vi "4155C Sample Config SMUs FPP v2.0.vi"(2 "FPP - Probe 2":u32(ring)=3 items=["SMU1  ", "SMU2  ", "SMU3  ", "SMU4  ", "SMU5  ", "SMU6  "], 4 "FPP - Probe 1":u32(ring) items=["SMU1  ", "SMU2  ", "SMU3  ", "SMU4  ", "SMU5  ", "SMU6  "], 5 "FPP - Drain":u32(ring)=1 items=["SMU1  ", "SMU2  ", "SMU3  ", "SMU4  ", "SMU5  ", "SMU6  "], 6 "FPP - Gate":u32(ring)=2 items=["SMU1  ", "SMU2  ", "SMU3  ", "SMU4  ", "SMU5  ", "SMU6  "], 7 "FPP - Source":u32(ring) items=["VSU1  ", "VSU2  "], 8 "error in (no error)":errorcluster, 9 "Drain Standby":bool, 10 "Gate Standby":bool, 11 "VISA resource name in":refnum<visa-resource-name>) -> (0 "error out":errorcluster, 3 "VISA Resource Name out":refnum<visa-resource-name>)   [LabVIEW 2016]
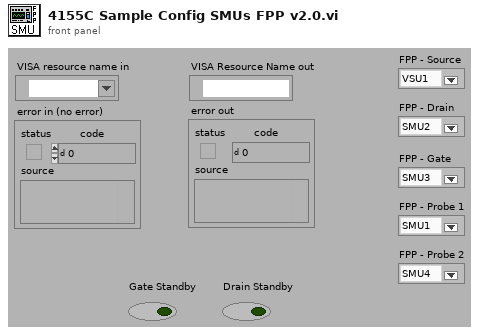
[diagram p1: front panel]
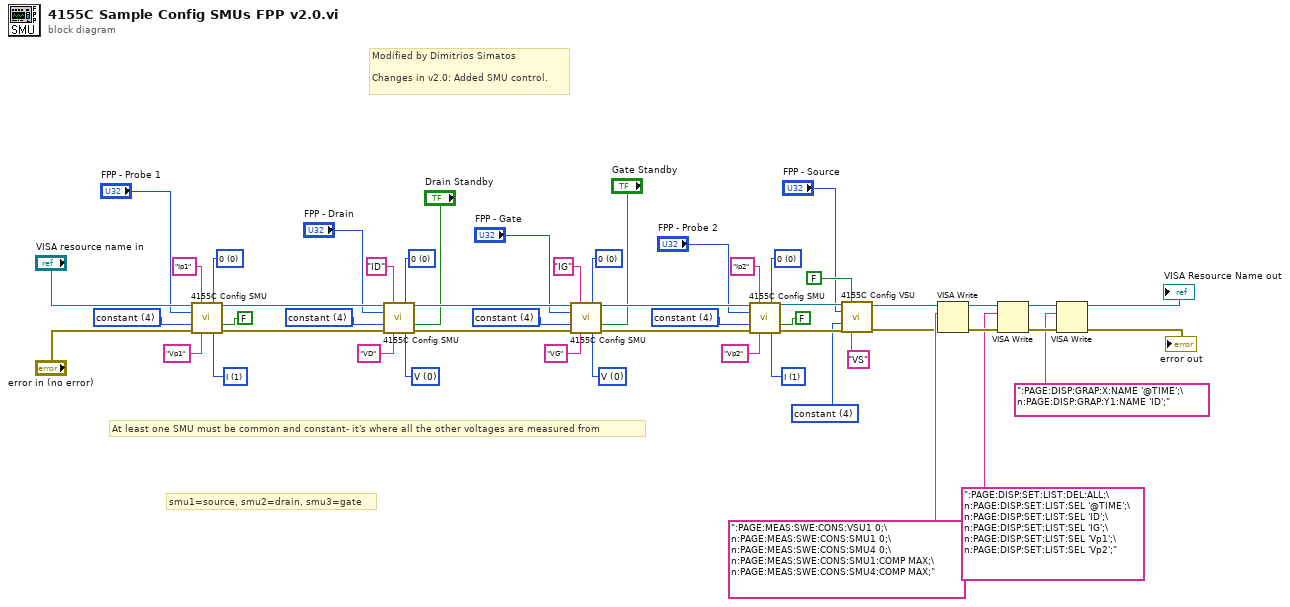
[diagram p0: block diagram]
diagram:
  w21 = u32 4 items=["disabled  ", "VAR1  ", "VAR2  ", "VAR1'  ", "constant  "] ("function")
  w32 = u32 1 items=["V  ", "I  ", "V pulse  ", "I pulse  ", "  common  "] ("mode")
  w33 = u32 0 items=["0  ", "10K Ohms  ", "100K Ohms  ", "1M Ohms  "] ("series resistance *")
  w35 = u32 4 items=["disabled  ", "VAR1  ", "VAR2  ", "VAR1'  ", "constant  "] ("function")
  w37 = u32 0 items=["V  ", "I  ", "V pulse  ", "I pulse  ", "  common  "] ("mode")
  w38 = u32 0 items=["0  ", "10K Ohms  ", "100K Ohms  ", "1M Ohms  "] ("series resistance *")
  w40 = u32 4 items=["disabled  ", "VAR1  ", "VAR2  ", "VAR1'  ", "constant  "] ("function")
  w42 = u32 0 items=["V  ", "I  ", "V pulse  ", "I pulse  ", "  common  "] ("mode")
  w43 = u32 0 items=["0  ", "10K Ohms  ", "100K Ohms  ", "1M Ohms  "] ("series resistance *")
  w45 = u32 4 items=["disabled  ", "VAR1  ", "VAR2  ", "VAR1'  ", "constant  "] ("function")
  w48 = u32 1 items=["V  ", "I  ", "V pulse  ", "I pulse  ", "  common  "] ("mode")
  w49 = u32 0 items=["0  ", "10K Ohms  ", "100K Ohms  ", "1M Ohms  "] ("series resistance *")
  w51 = u32 4 items=["disabled  ", "VAR1  ", "VAR2  ", "VAR1'  ", "constant  "] ("function")
  # "Modified by Dimitrios Simatos\n\nChanges in v2.0: Added SMU control."
  # "smu1=source, smu2=drain, smu3=gate"
  # "At least one SMU must be common and constant- it's where all the other voltages are measured from"
  n1 = call "4155C Config SMU.vi"("VISA session"="VISA resource name in", "I name (max 6 chars)"="Ip1", "series resistance *"=w49, "unit to configure"="FPP - Probe 1", "function"=w51, "standby"=FALSE, "error in (no error)"="error in (no error)", "V name (max 6 chars)"="Vp1", "mode"=w48) -> ("dup VISA resource name"=w29:refnum<visa-resource-name>, "error out"=w28:errorcluster)  [unwired: 5 in]
  n2 = call "4155C Config SMU.vi"("VISA session"=w29, "I name (max 6 chars)"="ID", "series resistance *"=w43, "unit to configure"="FPP - Drain", "function"=w45, "standby"="Drain Standby", "error in (no error)"=w28, "V name (max 6 chars)"="VD", "mode"=w42) -> ("dup VISA resource name"=w26:refnum<visa-resource-name>, "error out"=w27:errorcluster)  [unwired: 5 in]
  n3 = call "4155C Config SMU.vi"("VISA session"=w26, "I name (max 6 chars)"="IG", "series resistance *"=w38, "unit to configure"="FPP - Gate", "function"=w40, "standby"="Gate Standby", "error in (no error)"=w27, "V name (max 6 chars)"="VG", "mode"=w37) -> ("dup VISA resource name"=w25:refnum<visa-resource-name>, "error out"=w24:errorcluster)  [unwired: 5 in]
  n4 = call "4155C Config SMU.vi"("VISA session"=w25, "I name (max 6 chars)"="Ip2", "series resistance *"=w33, "unit to configure"="FPP - Probe 2", "function"=w35, "standby"=FALSE, "error in (no error)"=w24, "V name (max 6 chars)"="Vp2", "mode"=w32) -> ("dup VISA resource name"=w19:refnum<visa-resource-name>, "error out"=w23:errorcluster)  [unwired: 5 in]
  n5 = call "4155C Config VSU.vi"("VISA session"=w19, "standby"=FALSE, "unit to configure"="FPP - Source", "function"=w21, "error in (no error)"=w23, "V name (max 6 chars)"="VS") -> ("dup VISA resource name"=w16:refnum<visa-resource-name>, "error out"=w17:errorcluster)  [unwired: 8 in]
  n6 = VISA Write(VISA resource name=w16, write buffer=":PAGE:MEAS:SWE:CONS:VSU1 0;\n:PAGE:MEAS:SWE:CONS:SMU1 0;\n:PAGE:MEAS:SWE:CONS:SMU4 0;\n:PAGE:MEAS:SWE:CONS:SMU1:COMP MAX;\n:PAGE:MEAS:SWE:CONS:SMU4:COMP MAX;" ("write buffer (\"\")"), error in (no error)=w17) -> (VISA resource name out=w15:refnum<visa-resource-name>, error out=w10:errorcluster)  [unwired: 1 out]
  n7 = VISA Write(VISA resource name=w15, write buffer=":PAGE:DISP:SET:LIST:DEL:ALL;\n:PAGE:DISP:SET:LIST:SEL '@TIME';\n:PAGE:DISP:SET:LIST:SEL 'ID';\n:PAGE:DISP:SET:LIST:SEL 'IG';\n:PAGE:DISP:SET:LIST:SEL 'Vp1';\n:PAGE:DISP:SET:LIST:SEL 'Vp2';" ("write buffer (\"\")"), error in (no error)=w10) -> (VISA resource name out=w14:refnum<visa-resource-name>, error out=w11:errorcluster)  [unwired: 1 out]
  n8 = VISA Write(VISA resource name=w14, write buffer=":PAGE:DISP:GRAP:X:NAME '@TIME';\n:PAGE:DISP:GRAP:Y1:NAME 'ID';" ("write buffer (\"\")"), error in (no error)=w11) -> (VISA resource name out=→"VISA Resource Name out":refnum<visa-resource-name>, error out=→"error out":errorcluster)  [unwired: 1 out]
